vi "show_color_xyz_from_loaded spectra.vi"() -> ()   [LabVIEW 2022 SP3]
uses:
  <vilib>/Utility/file.llb/Read From Spreadsheet File (DBL).vi
panel:
  out "Waveform Graph":dbl[](graph)
  out "z":dbl
  out "y":dbl
  out "x":dbl
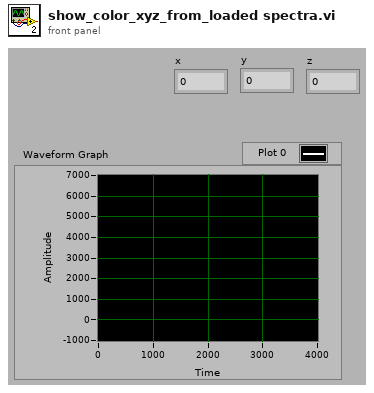
[diagram p1: front panel]
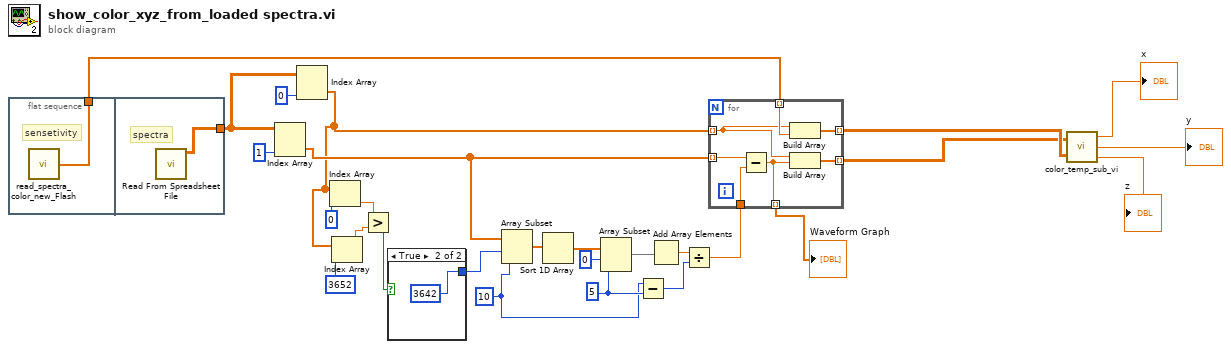
[diagram p0: block diagram]
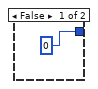
[diagram p2: hidden frame]
diagram:
  w20 = 5 ("length")
  w19 = 10 ("length")
  n1 = flat-sequence {
    tunnel: [w28] -> w10
    tunnel: [w29] -> w12
    frame #0 {
      # "sensetivity"
      n2 = call "read_spectra_color_new_Flash.vi"() -> ("correction"=w28:dbl[])
    }
    frame #1 {
      # "spectra"
      n3 = call-poly <vilib>:"Read From Spreadsheet File.vi"() -> ("all rows"=w29:dbl[][])  [unwired: 7 in, 4 out]
    }
  }
  n4 = Index Array(array=w12, index (col)=1 ("disabled index (col)")) -> (element=w3:dbl[])  [unwired: 1 in]
  n5 = Index Array(array=w12, index (col)=0 ("disabled index (col)")) -> (element=w2:dbl[])  [unwired: 1 in]
  n6 = Index Array(array=w2, index=0) -> (element=w16:dbl)
  n7 = Index Array(array=w2, index=3652) -> (element=w15:dbl)
  n8 = Greater?(x=w16, y=w15) -> (0:w21:bool)
  n9 = case shown="True" w21 {
    tunnel: [0 ("index") 3642] -> w18
    frame False {
    }
    frame True {
    }
  }
  n10 = Array Subset(array=w3, index=w18, length=w19) -> (w4:dbl[])
  n11 = Sort 1D Array(array=w4) -> (sorted array=w27:dbl[])
  n12 = Array Subset(array=w27, index=0, length=w20) -> (w26:dbl[])
  n13 = Subtract(x=w19, y=w20) -> (x-y=w24:i32)
  n14 = Add Array Elements(numeric array=w26) -> (sum=w25:dbl)
  n15 = Divide(x=w25, y=w24) -> (x/y=w11:dbl)
  n16 = for {
    tunnel: w11 -> [w38]
    tunnel: w3 -> [w37] mode=indexing
    tunnel: w10 -> [w36] mode=indexing
    tunnel: w2 -> [w35] mode=indexing
    tunnel: [w34] -> w9 mode=indexing
    tunnel: [w33] -> w8 mode=indexing
    tunnel: [w32] -> w1 mode=indexing
    n17 = Subtract(x=w37, y=w38) -> (x-y=w32:dbl)
    n18 = Build Array(w35, w36) -> (w34:dbl[])
    n19 = Build Array(w35, w32) -> (w33:dbl[])
  }
  "Waveform Graph" <- w1
  n20 = call "color_temp_sub_vi.vi"("spectra"=w8, "sensesitivity"=w9) -> ("x"=→"x":dbl, "y"=→"y":dbl, "z"=→"z":dbl)
